vi "what_do_you_want_end.vi"() -> (0 "Log out":bool)   [LabVIEW 2014]
panel:
  in  "Cluster":cluster{"OK Button 2":bool, "stop":bool}
  # "Your booking is compelete.\nWhat do you want to do now?\n1.Buy more movie ticket.\n2.Log out."
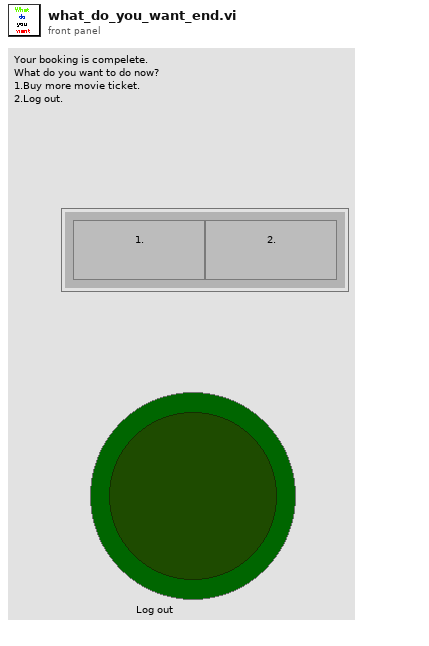
[diagram p1: front panel]
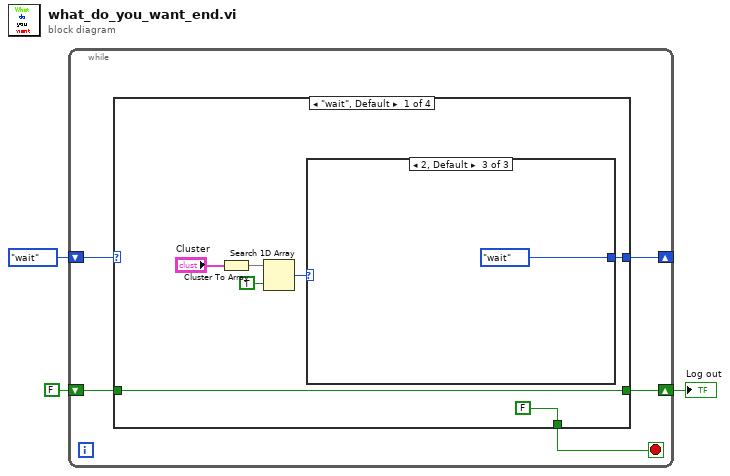
[diagram p0: block diagram]
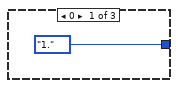
[diagram p2: hidden frame]
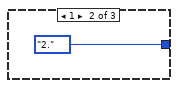
[diagram p3: hidden frame]
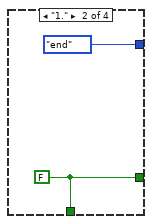
[diagram p4: hidden frame]
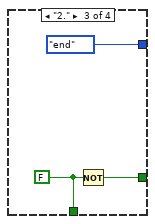
[diagram p5: hidden frame]
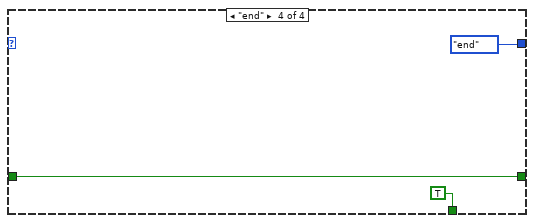
[diagram p6: hidden frame]
diagram:
  n1 = while {
    shift-right: [w7] -> _
    shift-left: enum16{"wait", "1.", "2.", "3.", "end"}."wait" -> [w8]
    shift-right: [w5] -> w2
    shift-left: FALSE -> [w4]
    stop <- w6 stop-if-true
    n2 = case shown="\"wait\", Default" w8 {
      tunnel: [w11 enum16{"wait", "1.", "2.", "3.", "end"}."end" enum16{"wait", "1.", "2.", "3.", "end"}."end" enum16{"wait", "1.", "2.", "3.", "end"}."end"] -> w7
      tunnel: [FALSE w19 w22 TRUE] -> w6
      tunnel: [w9 w19 w21 w24] -> w5
      tunnel: w4 -> [w9 _ _ w24]
      frame "wait", Default {
        n3 = Cluster To Array(cluster="Cluster") -> (array=w14:bool[])
        n4 = Search 1D Array(1D array=w14, element=TRUE) -> (index of element=w12:i32)  [unwired: 1 in]
        n5 = case shown="2, Default" w12 {
          tunnel: [enum16{"wait", "1.", "2.", "3.", "end"}."1." enum16{"wait", "1.", "2.", "3.", "end"}."2." enum16{"wait", "1.", "2.", "3.", "end"}."wait"] -> w11
          frame 0 {
          }
          frame 1 {
          }
          frame 2, Default {
          }
        }
      }
      frame "1." {
        w19 = FALSE
      }
      frame "2." {
        w22 = FALSE
        n6 = Not(x=w22) -> (.not. x?=w21:bool)
      }
      frame "end" {
      }
    }
  }
  "Log out" <- w2
